vi "BuildDIOtask.vi"(8 "error in (no error)":errorcluster, 9 "Input Cluster":T2, 10 "skipped outbit chans (7)":i32, 11 "Task cluster in":T1={"inbits"=8, "outbits"=38, "Counter"="", "Inbits"="", "Outbits"="", "Fast AO"=[], "Errors"={"status"=FALSE, "code"=0, "source"=""}}) -> (2 "Task cluster out":T1={"inbits"=8, "outbits"=38, "Counter"="", "Inbits"="", "Outbits"="", "Fast AO"=[], "Errors"={"status"=FALSE, "code"=0, "source"=""}}, 3 "counter trig":tag)   [LabVIEW 2018]
uses:
  Tasks_RT.ctl
  <vilib>/DAQmx/create/channels.llb/DAQmx Create Channel (DI-Digital Input).vi
  <vilib>/DAQmx/create/channels.llb/DAQmx Create Channel (DO-Digital Output).vi
  <resource>/objmgr/daqmx.rc
panel:
  # "Tasks and errors"
  # "Tasks and errors"
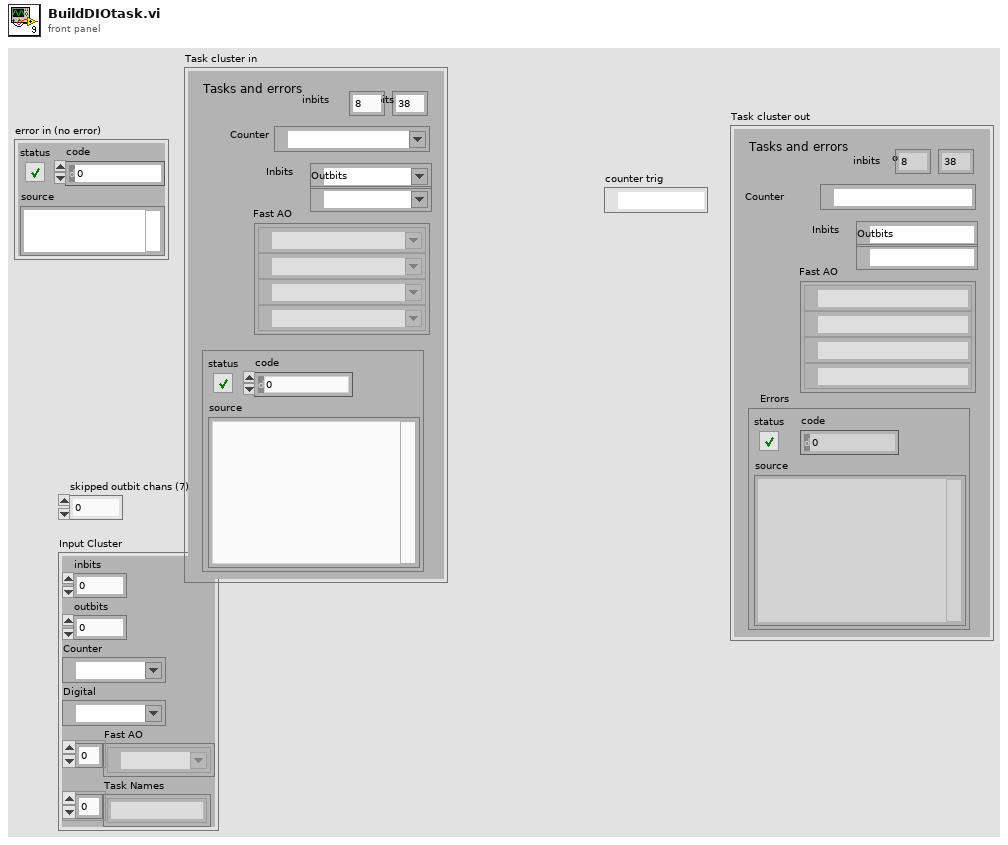
[diagram p1: front panel]
types:
  T1 = typedef "Tasks_RT.ctl" = cluster{"inbits":i32, "outbits":i32, "Counter":refnum<k21>, "Inbits":refnum<k21>, "Outbits":refnum<k21>, "Fast AO":refnum<k21>[], "Errors":errorcluster}
  T2 = cluster{"inbits":i32, "outbits":i32, "Counter":tag, "Digital":tag, "Fast AO":tag[], "Task Names":string[]}
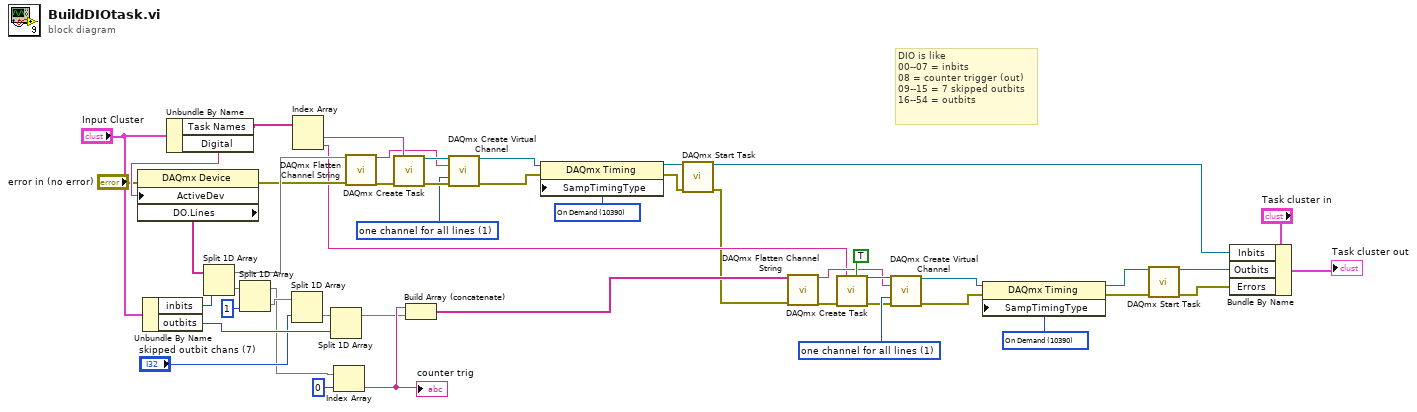
[diagram p0: block diagram]
diagram:
  w13 = 1 items=["one channel for each line", "one channel for all lines"] ("line grouping")
  w17 = 10390 items=["Sample Clock"=10388, "Burst Handshake"=12548, "Handshake"=10389, "Implicit"=10451, "On Demand"=10390, "Change Detection"=12504, "Pipelined Sample Clock"=14668] ("SampTimingType")
  w33 = 1 items=["one channel for each line", "one channel for all lines"] ("line grouping")
  w25 = 10390 items=["Sample Clock"=10388, "Burst Handshake"=12548, "Handshake"=10389, "Implicit"=10451, "On Demand"=10390, "Change Detection"=12504, "Pipelined Sample Clock"=14668] ("SampTimingType")
  # "DIO is like\n00--07 = inbits\n08 = counter trigger (out)\n09--15 = 7 skipped outbits\n16--54 = outbits"
  n1 = Unbundle By Name("Input Cluster") -> ("inbits"=w38:i32, "outbits"=w45:i32)
  n2 = Unbundle By Name("Input Cluster") -> ("Task Names"=w32:string[], "Digital"=w22:tag)
  n3 = property class="DAQmx Device"(error in="error in (no error)", "ActiveDev"=w22) -> (error out=w11:errorcluster, "DO.Lines"=w36:tag[])  [unwired: 1 in, 1 out]
  n4 = Split 1D Array(array=w36, index=w38) -> (first subarray=w12:tag[], second subarray=w39:tag[])
  n5 = Split 1D Array(array=w39, index=1) -> (first subarray=w40:tag[], second subarray=w42:tag[])
  n6 = Split 1D Array(array=w42, index="skipped outbit chans (7)") -> (second subarray=w44:tag[])  [unwired: 1 out]
  n7 = Index Array(array=w32) -> (element #1=w10:string, element #2=w9:string)  [unwired: 2 in]
  n8 = Split 1D Array(array=w44, index=w45) -> (first subarray=w46:tag[])  [unwired: 1 out]
  n9 = Index Array(array=w40, index=0) -> (element=w47:tag)
  "counter trig" <- w47
  n10 = call <vilib>:"DAQmx Flatten Channel String.vi"("names in"=w12, "error in"=w11) -> ("names out"=w6:string, "error out"=w15:errorcluster)  [unwired: 12 in]
  n11 = call <vilib>:"DAQmx Create Task.vi"("new task name"=w10, "error in"=w15) -> ("task out"=w14:refnum<k21>, "error out"=w16:errorcluster)  [unwired: 12 in]
  n12 = Build Array (concatenate)(w47, w46) -> (w48:tag[])
  n13 = call-poly <vilib>:"DAQmx Create Virtual Channel.vi"("task in"=w14, "lines"=w6, "line grouping"=w13, "error in"=w16) -> ("task out"=w19:refnum<k21>, "error out"=w18:errorcluster)  [unwired: 10 in]
  n14 = property class="DAQmx Timing"(reference=w19, error in=w18, "SampTimingType"=w17) -> (reference out=w5:refnum<k21>, error out=w4:errorcluster)
  n15 = call <vilib>:"DAQmx Start Task.vi"("task/channels in"=w5, "error in"=w4) -> ("task out"=w7:refnum<k21>, "error out"=w3:errorcluster)  [unwired: 12 in]
  n16 = call <vilib>:"DAQmx Flatten Channel String.vi"("names in"=w48, "error in"=w3) -> ("names out"=w28:string, "error out"=w27:errorcluster)  [unwired: 12 in]
  n17 = call <vilib>:"DAQmx Create Task.vi"("new task name"=w9, "auto cleanup"=TRUE, "error in"=w27) -> ("task out"=w29:refnum<k21>, "error out"=w26:errorcluster)  [unwired: 11 in]
  n18 = call-poly <vilib>:"DAQmx Create Virtual Channel.vi"("task in"=w29, "lines"=w28, "line grouping"=w33, "error in"=w26) -> ("task out"=w23:refnum<k21>, "error out"=w24:errorcluster)  [unwired: 10 in]
  n19 = property class="DAQmx Timing"(reference=w23, error in=w24, "SampTimingType"=w25) -> (reference out=w34:refnum<k21>, error out=w35:errorcluster)
  n20 = call <vilib>:"DAQmx Start Task.vi"("task/channels in"=w34, "error in"=w35) -> ("task out"=w8:refnum<k21>, "error out"=w2:errorcluster)  [unwired: 12 in]
  n21 = Bundle By Name(cluster="Task cluster in", "Inbits"=w7, "Outbits"=w8, "Errors"=w2) -> (→"Task cluster out":T1)
